vi "Q_AllTotal.vi"(8 "error in (no error)":errorcluster, 11 "Data Manager in":refnum<class "Data Manager.lvclass">) -> (0 "error out":errorcluster, 1 "Total Target":dbl, 2 "Total Travelled":dbl, 3 "Data Manager out":refnum<class "Data Manager.lvclass">)   [LabVIEW 2020, in "Data Manager.lvclass"]
uses:
  Data Manager.lvclass
  Data Manager.lvclass/Data Manager.ctl
  <vilib>/drjdpowell/SQLite Library/SQL Connection/Execute SQL (DBL results).vi
  <vilib>/drjdpowell/SQLite Library/SQLite.lvlib
  <vilib>/drjdpowell/SQLite Library/SQL Connection/Connection.lvclass
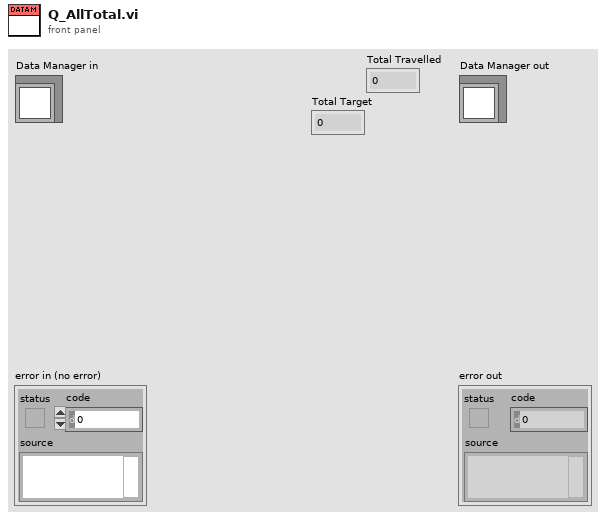
[diagram p1: front panel]
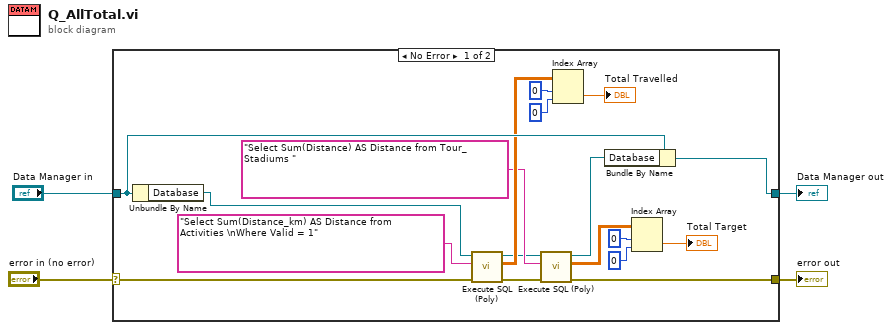
[diagram p0: block diagram]
diagram:
  n1 = case shown="No Error" "error in (no error)" {
    selector: "error in (no error)" -> [w19 w24]
    tunnel: [w12 w24] -> w3
    tunnel: [w20 w23] -> w1
    tunnel: "Data Manager in" -> [w21 w23]
    frame No Error {
      n2 = Unbundle By Name(w21) -> ("Database"=w22:refnum<class "Connection.lvclass">)
      n3 = call-poly <vilib>:"Execute SQL (Poly).vi"("error in (no error)"=w19, "SQL"="Select Sum(Distance_km) AS Distance from Activities \nWhere Valid = 1", "SQLite Connection in"=w22) -> ("error out"=w13:errorcluster, "Result Set"=w17:dbl[][], "SQLite Connection"=w10:refnum<class "Connection.lvclass">)  [unwired: 5 in, 1 out]
      n4 = call-poly <vilib>:"Execute SQL (Poly).vi"("error in (no error)"=w13, "SQL"="Select Sum(Distance) AS Distance from Tour_Stadiums ", "SQLite Connection in"=w10) -> ("error out"=w12:errorcluster, "Result Set"=w6:dbl[][], "SQLite Connection"=w9:refnum<class "Connection.lvclass">)  [unwired: 5 in, 1 out]
      n5 = Index Array(array=w17, index (row)=0 ("disabled index (row)"), index (col)=0 ("disabled index (col)")) -> (element=→"Total Travelled":dbl)
      n6 = Bundle By Name(cluster=w21, "Database"=w9) -> (w20:refnum<class "Data Manager.lvclass">)
      n7 = Index Array(array=w6, index (row)=0 ("disabled index (row)"), index (col)=0 ("disabled index (col)")) -> (element=→"Total Target":dbl)
    }
    frame Error {
    }
  }
  "error out" <- w3
  "Data Manager out" <- w1
